vi "init_34450.vi"(8 "Rozsah 3450A":T1(ring), 9 "Rozliseni 34450":enum16{"4_1/2 fast", "4_1/2 slow", "5_1/2 fast"}(ring), 10 "Pocet mereni na prumer":u32=1 min=1 max=20, 11 "Pocet mereni za sekundu":u32=1 min=1 max=5) -> (2 "Command String":string)   [LabVIEW 2021]
panel:
  # "34450 - VOLTMETR"
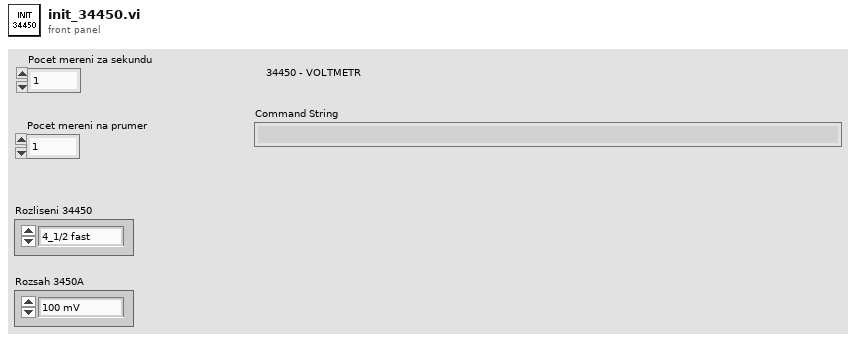
[diagram p1: front panel]
types:
  T1 = enum16{"100 mV", "1 V", "10 V", "100 V", "1000 V"}
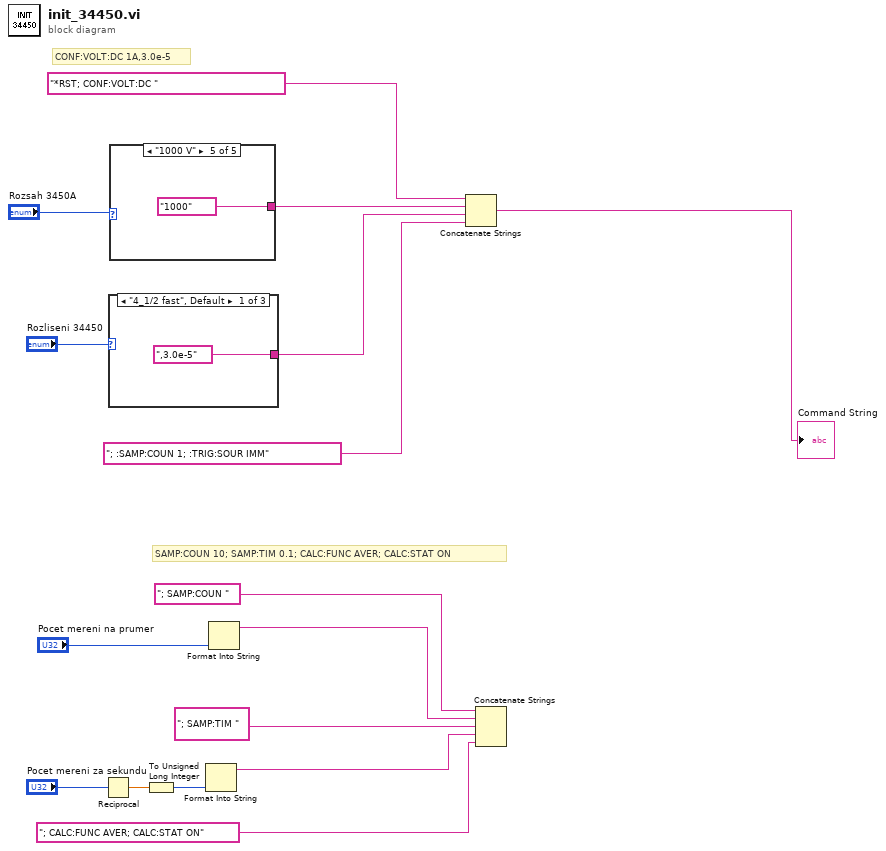
[diagram p0: block diagram]
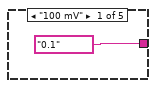
[diagram p2: hidden frame]
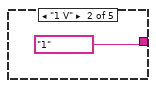
[diagram p3: hidden frame]
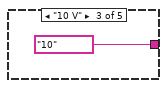
[diagram p4: hidden frame]
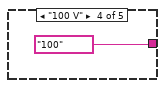
[diagram p5: hidden frame]
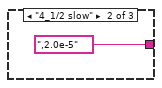
[diagram p6: hidden frame]
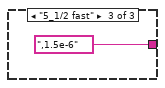
[diagram p7: hidden frame]
diagram:
  # "SAMP:COUN 10; SAMP:TIM 0.1; CALC:FUNC AVER; CALC:STAT ON"
  # "CONF:VOLT:DC 1A,3.0e-5"
  n1 = Reciprocal(x="Pocet mereni za sekundu") -> (1/x=w10:dbl)
  n2 = case shown="\"4_1/2 fast\", Default" "Rozliseni 34450" {
    tunnel: [",3.0e-5" ",2.0e-5" ",1.5e-6"] -> w13
    frame "4_1/2 fast", Default {
    }
    frame "4_1/2 slow" {
    }
    frame "5_1/2 fast" {
    }
  }
  n3 = case shown="\"1000 V\"" "Rozsah 3450A" {
    tunnel: ["0.1" "1" "10" "100" "1000"] -> w14
    frame "100 mV" {
    }
    frame "1 V" {
    }
    frame "10 V" {
    }
    frame "100 V" {
    }
    frame "1000 V" {
    }
  }
  n4 = To Unsigned Long Integer(number=w10) -> (unsigned 32bit integer=w9:u32)
  n5 = Format Into String(w9) -> (resulting string=w5:string)  [unwired: 3 in, 1 out]
  n6 = Format Into String("Pocet mereni na prumer") -> (resulting string=w7:string)  [unwired: 3 in, 1 out]
  n7 = Concatenate Strings("*RST; CONF:VOLT:DC ", w14, w13, "; :SAMP:COUN 1; :TRIG:SOUR IMM") -> (→"Command String":string)
  n8 = Concatenate Strings("; SAMP:COUN ", w7, "; SAMP:TIM ", w5, "; CALC:FUNC AVER; CALC:STAT ON") -> ()  [unwired: 1 out]
